vi "GetAllPropertiesValues.vi"(8 "error in (no error)":errorcluster, 11 "CSSProperties in":refnum<class "CSSProperties.lvclass">) -> (0 "error out":errorcluster, 2 "KVPs":cluster{"Properties":string, "Values":string}[](array[cluster]), 3 "CSSProperties out":refnum<class "CSSProperties.lvclass">)   [LabVIEW 2019, in "CSSProperties.lvclass"]
uses:
  CSSProperties.lvclass
  CSSProperties.lvclass/CSSProperties.ctl
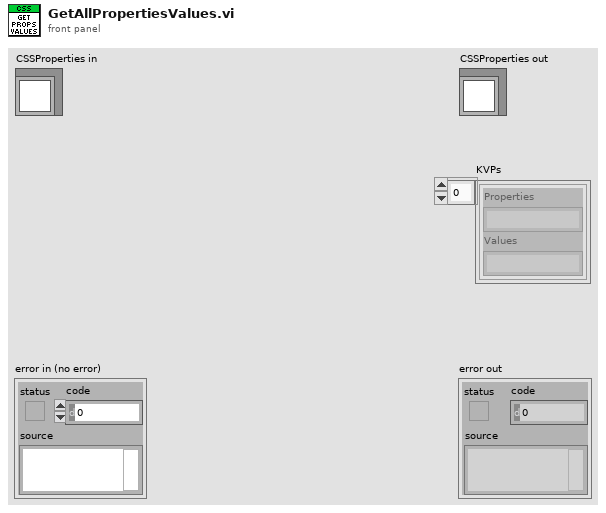
[diagram p1: front panel]
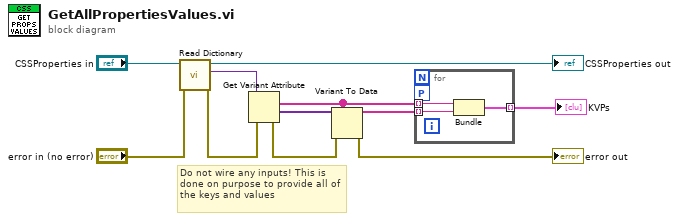
[diagram p0: block diagram]
diagram:
  # "Do not wire any inputs! This is done on purpose to provide all of the keys and values"
  n1 = call "Read Dictionary.vi"("error in (no error)"="error in (no error)", "CSSProperties in"="CSSProperties in") -> ("error out"=w3:errorcluster, "Dictionary"=w4:variant, "CSSProperties out"=→"CSSProperties out":refnum<class "CSSProperties.lvclass">)  [unwired: 7 in]
  n2 = Get Variant Attribute(Variant=w4, error in=w3) -> (names=w7:string[], values=w9:variant[], error out=w2:errorcluster)  [unwired: 2 in, 1 out]
  n3 = Variant To Data(error in=w2, type=w7, Variant=w9) -> (data=w8:string[], error out=→"error out":errorcluster)
  n4 = for {
    tunnel: w8 -> [w13] mode=indexing
    tunnel: w7 -> [w14] mode=indexing
    tunnel: [w12] -> w5 mode=indexing
    workers-P: _ -> [_]
    n5 = Bundle(w14, w13) -> (w12:cluster{string, string})  [unwired: 1 in]
  }
  "KVPs" <- w5
